vi "Execute.GetStatusChannels.vi"(8 "error in (no error)":errorcluster, 10 "Cluster":T1={"NIVS.BaseLogPath"=path "", "NIVS.SystemDefinitionFile"=path "", "NIVS.Events"={"SequenceEvent"=refnum, "SystemChangeEvent"=refnum, "WorkspaceEvent"=refnum}, "NIVS.SequenceState"=enum."Idle", "NIVS.GatewayIPAddress"="", "NIVS.DataLogSpecRef"=refnum, "NIVS.DataLogManagerRef"=refnum, "NIVS.LogSessionGUID"="", "NIVS.WorkspaceManager"=refnum, "NIVS.Deployed"=FALSE, "NIVS.ProfileRef"=refnum, "NIVS.ProfileCallback"=refnum, "NIVS.SystemStateRefs"={"CustDatRef"=refnum, "EvtRef"=refnum}, "UI.Abort"=refnum, "UI.Pause"=refnum, "UI.EnableLogging"=refnum, "UI.Start"=refnum, "UI.LogChannels"=refnum, "UI.StartIteration"=refnum, "UI.StartStep"=refnum, "UI.Sequence"=refnum, "UI.PreviewMode"=refnum, "UI.Graph"=refnum, "UI.BaseFileName"=refnum, "UI.Profiles"=refnum, "UI.CurrentStep"=refnum, "UI.CurrentIteration"=refnum, "UI.TotalIterations"=refnum, "Sequence.AbortChannel"="", "Sequence.StepInfoChannel"="", "Sequence.Iterations"=0, "Sequence.IterationInfoChannel"="", "Sequence.#ofColumns"=0, "Events.State"=refnum, "Events.Test Result"=refnum, "Events.Progress"=refnum, "INI.Settings"={"Build Location"=path "C:/Simple Sequence Editor/SequenceRepo", "LoggingLocation"=path ""}}, 11 "Commands":string[](array[string])) -> (0 "error out":errorcluster, 3 "Commands out":string[](array[string]))   [LabVIEW 2013, in "Simple Sequence Tools - Execution.lvlib"]
uses:
  Simple Sequence Tools - Execution.lvlib
  Types/Main.StateVariables.ctl
  Types/Execute.UserEventRefs.ctl
  <vilib>/NI Veristand/Execution/Workspace/SystemStateRegEventRef.ctl
  Types/Execution.SequenceState.ctl
  <vilib>/NI Veristand/Execution/DataLogging/DataLoggingSpecification Ref.ctl
  NationalInstruments.VeriStand.ClientAPI
  <vilib>/NI Veristand/Execution/DataLogging/IDataLogging Ref.ctl
  <vilib>/NI Veristand/Execution/Workspace/WorkspaceAPI.ctl
  NationalInstruments.VeriStand.RealTimeSequenceDefinitionApi
  <vilib>/NI Veristand/Execution/Workspace/SystemStateEventRef.ctl
  Shared/Types/INI.Settings
  <vilib>/NI Veristand/Execution/Workspace/NI VeriStand - Get Single Channel Value.vi
  <vilib>/NI Veristand/Execution/Workspace/NI_VS Workspace ExecutionAPI.lvlib
  <vilib>/NI Veristand/Execution/DataLogging/NI_VS Data Logging API.lvlib
  Shared/Simple Sequence Tools - Shared.lvlib
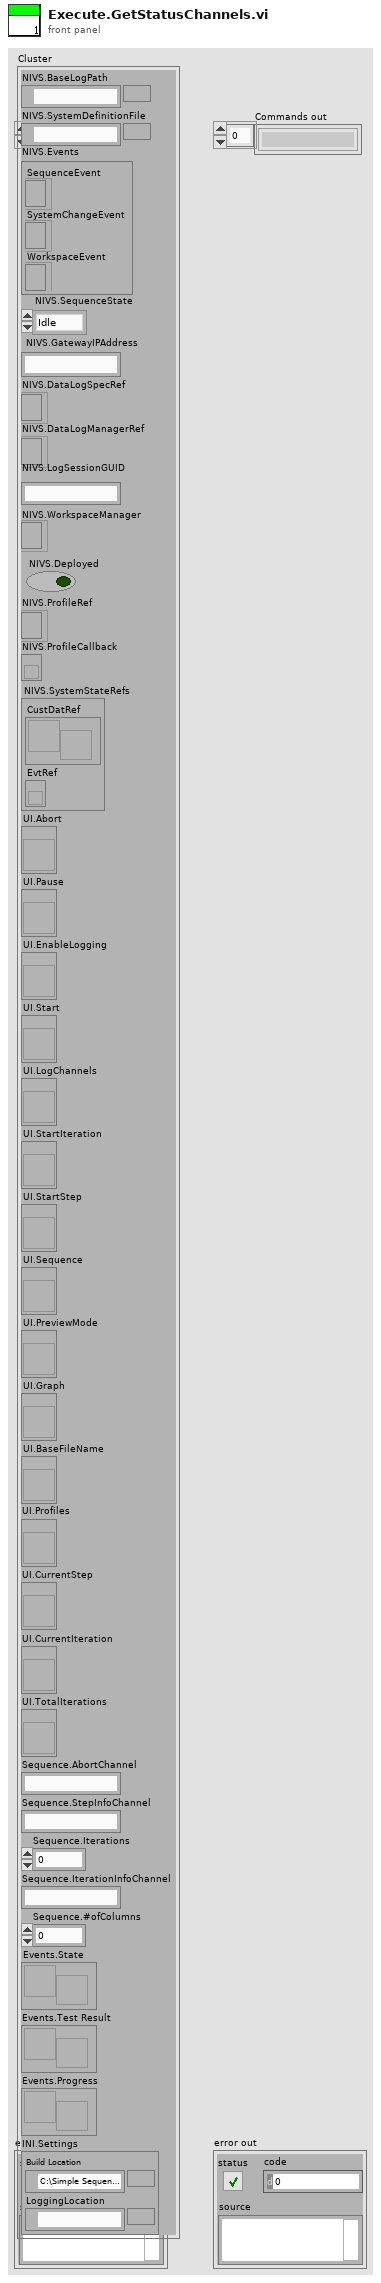
[diagram p1: front panel]
types:
  T1 = typedef "Simple Sequence Tools - Execution.lvlib/Main.StateVariables.ctl" = cluster{"NIVS.BaseLogPath":path, "NIVS.SystemDefinitionFile":path, "NIVS.Events":T2, "NIVS.SequenceState":T4, "NIVS.GatewayIPAddress":string, "NIVS.DataLogSpecRef":T5, "NIVS.DataLogManagerRef":T6, "NIVS.LogSessionGUID":string, "NIVS.WorkspaceManager":T7, "NIVS.Deployed":bool, "NIVS.ProfileRef":refnum<k24>, "NIVS.ProfileCallback":refnum<k27>, "NIVS.SystemStateRefs":T8, "UI.Abort":refnum<vi>, "UI.Pause":refnum<vi>, "UI.EnableLogging":refnum<vi>, "UI.Start":refnum<vi>, "UI.LogChannels":refnum<vi>, "UI.StartIteration":refnum<vi>, "UI.StartStep":refnum<vi>, "UI.Sequence":refnum<vi>, "UI.PreviewMode":refnum<vi>, "UI.Graph":refnum<vi>, "UI.BaseFileName":refnum<vi>, "UI.Profiles":refnum<vi>, "UI.CurrentStep":refnum<vi>, "UI.CurrentIteration":refnum<vi>, "UI.TotalIterations":refnum<vi>, "Sequence.AbortChannel":string, "Sequence.StepInfoChannel":string, "Sequence.Iterations":u32, "Sequence.IterationInfoChannel":string, "Sequence.#ofColumns":i32, "Events.State":refnum<user-event>, "Events.Test Result":refnum<user-event>, "Events.Progress":refnum<user-event>, "INI.Settings":T9}
  T2 = typedef "Simple Sequence Tools - Execution.lvlib/Execute.UserEventRefs.ctl" = cluster{"SequenceEvent":refnum<event-registration>, "SystemChangeEvent":T3, "WorkspaceEvent":refnum<event-registration>}
  T3 = typedef "NI_VS Workspace ExecutionAPI.lvlib/SystemStateRegEventRef.ctl" = refnum<event-registration>
  T4 = typedef "Simple Sequence Tools - Execution.lvlib/Execution.SequenceState.ctl" = enum16{"Idle", "Initializing", "Running", "Paused", "Finalizing", "Complete"}
  T5 = typedef "NI_VS Data Logging API.lvlib/DataLoggingSpecification Ref.ctl" = refnum<k24>
  T6 = typedef "NI_VS Data Logging API.lvlib/IDataLogging Ref.ctl" = refnum<k24>
  T7 = typedef "NI_VS Workspace ExecutionAPI.lvlib/WorkspaceAPI.ctl" = refnum<k24>
  T8 = typedef "NI_VS Workspace ExecutionAPI.lvlib/SystemStateEventRef.ctl" = cluster{"CustDatRef":refnum<user-event>, "EvtRef":refnum<k27>}
  T9 = typedef "Simple Sequence Tools - Shared.lvlib/INI.Settings" = cluster{"Build Location":path, "LoggingLocation":path}
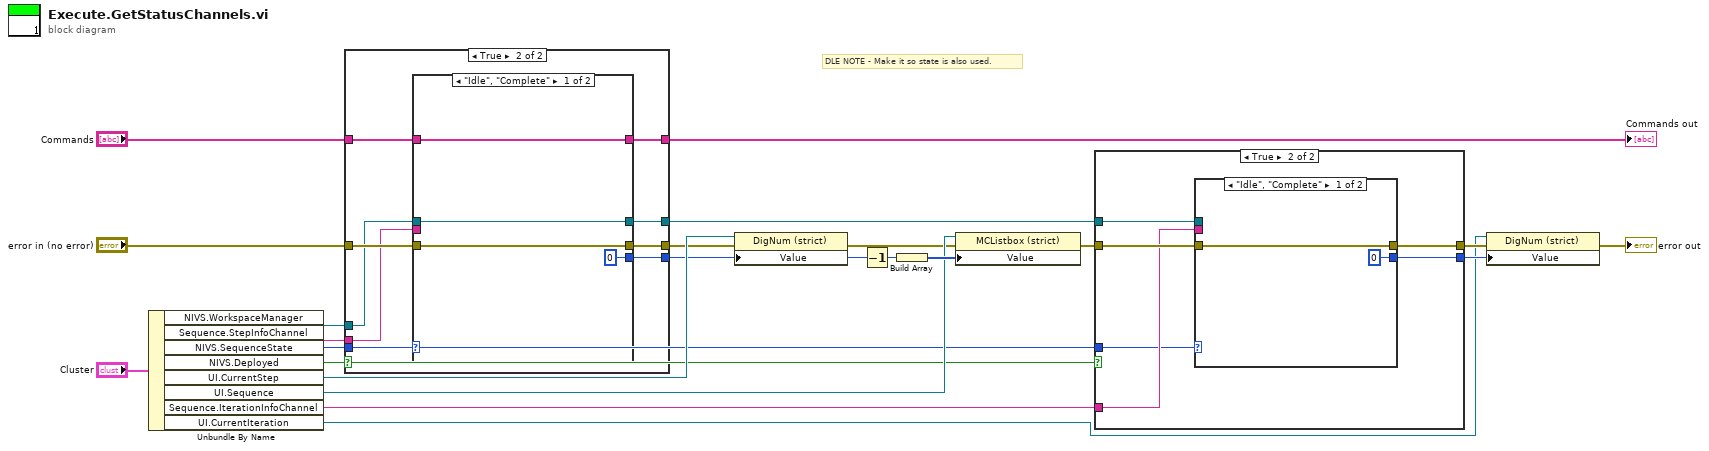
[diagram p0: block diagram]
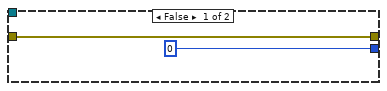
[diagram p2: hidden frame]
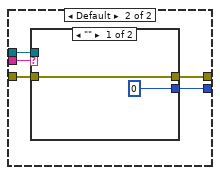
[diagram p3: hidden frame]
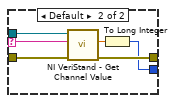
[diagram p4: hidden frame]
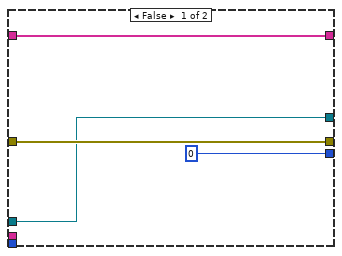
[diagram p5: hidden frame]
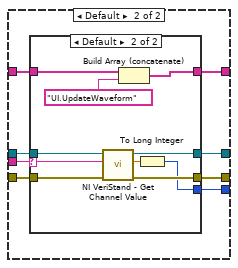
[diagram p6: hidden frame]
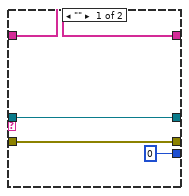
[diagram p7: hidden frame]
diagram:
  # "DLE NOTE - Make it so state is also used."
  n1 = Unbundle By Name("Cluster") -> ("NIVS.WorkspaceManager"=w14:T7, "Sequence.StepInfoChannel"=w16:string, "NIVS.SequenceState"=w1:T4, "NIVS.Deployed"=w7:bool, "UI.CurrentStep"=w11:refnum<vi>, "UI.Sequence"=w12:refnum<vi>, "Sequence.IterationInfoChannel"=w21:string, "UI.CurrentIteration"=w3:refnum<vi>)
  n2 = case shown="True" w7 {
    tunnel: w14 -> [w23 w33]
    tunnel: "error in (no error)" -> [w26 w35]
    tunnel: [w26 w34] -> w9
    tunnel: w16 -> [_ w31]
    tunnel: [0 w32] -> w8
    tunnel: "Commands" -> [w24 w30]
    tunnel: [w24 w29] -> w19
    tunnel: [w23 w28] -> w20
    tunnel: w1 -> [_ w27]
    frame False {
    }
    frame True {
      n3 = case shown="\"Idle\", \"Complete\"" w27 {
        tunnel: w35 -> [w37 w47]
        tunnel: [w37 w46] -> w34
        tunnel: w33 -> [w38 w45]
        tunnel: [0 w44] -> w32
        tunnel: w31 -> [_ w43]
        tunnel: w30 -> [w39 w42]
        tunnel: [w39 w41] -> w29
        tunnel: [w38 w40] -> w28
        frame "Idle", "Complete" {
        }
        frame Default {
          n4 = case shown="Default" w43 {
            selector: w43 -> [_ w56]
            tunnel: w47 -> [w51 w61]
            tunnel: [w51 w60] -> w46
            tunnel: w45 -> [w48 w59]
            tunnel: [0 w57] -> w44
            tunnel: w42 -> [w49 w54]
            tunnel: [w49 w53] -> w41
            tunnel: [w48 w52] -> w40
            frame "" {
            }
            frame Default {
              n5 = call-poly <vilib>:"NI VeriStand - Get Channel Value.vi"("error in (no error)"=w61, "Channel"=w56, "WorkspaceManager in"=w59) -> ("error out"=w60:errorcluster, "Value"=w58:dbl, "WorkspaceManager out"=w52:T7)  [unwired: 6 in]
              n6 = Build Array (concatenate)(w54, "UI.UpdateWaveform") -> (w53:string[])
              n7 = To Long Integer(number=w58) -> (32bit integer=w57:i32)
            }
          }
        }
      }
    }
  }
  "Commands out" <- w19
  n8 = property class="DigNum (strict)"(reference=w11, error in=w9, "Value"=w8) -> (error out=w10:errorcluster)  [unwired: 1 out]
  n9 = Decrement(x=w8) -> (x-1=w2:i32)
  n10 = Build Array(w2) -> (w17:i32[])
  n11 = property class="MCListbox (strict)"(reference=w12, error in=w10, "Value"=w17) -> (error out=w22:errorcluster)  [unwired: 1 out]
  n12 = case shown="True" w7 {
    tunnel: w20 -> [_ w67]
    tunnel: w22 -> [w63 w69]
    tunnel: [w63 w68] -> w5
    tunnel: w21 -> [_ w65]
    tunnel: [0 w66] -> w4
    tunnel: w1 -> [_ w64]
    frame False {
    }
    frame True {
      n13 = case shown="\"Idle\", \"Complete\"" w64 {
        tunnel: w69 -> [w71 w76]
        tunnel: [w71 w75] -> w68
        tunnel: w67 -> [_ w74]
        tunnel: [0 w73] -> w66
        tunnel: w65 -> [_ w72]
        frame "Idle", "Complete" {
        }
        frame Default {
          n14 = case shown="\"\"" w72 {
            selector: w72 -> [_ w79]
            tunnel: w76 -> [w78 w84]
            tunnel: [w78 w83] -> w75
            tunnel: w74 -> [_ w82]
            tunnel: [0 w80] -> w73
            frame "" {
            }
            frame Default {
              n15 = call-poly <vilib>:"NI VeriStand - Get Channel Value.vi"("error in (no error)"=w84, "Channel"=w79, "WorkspaceManager in"=w82) -> ("error out"=w83:errorcluster, "Value"=w81:dbl)  [unwired: 6 in, 1 out]
              n16 = To Long Integer(number=w81) -> (32bit integer=w80:i32)
            }
          }
        }
      }
    }
  }
  n17 = property class="DigNum (strict)"(reference=w3, error in=w5, "Value"=w4) -> (error out=→"error out":errorcluster)  [unwired: 1 out]
